vi "Configure.vi"(8 "error in (no error)":errorcluster caption="错误输入（无错误）", 11 "34401A 输入":refnum<class "34401A.lvclass">) -> (0 "error out":errorcluster caption="错误输出", 3 "34401A 输出":refnum<class "34401A.lvclass">)   [LabVIEW 2020, in "34401A.lvlib" / "34401A.lvclass"]
uses:
  34401A.lvclass
  <instrlib>/Agilent 34401/Agilent 34401.lvlib
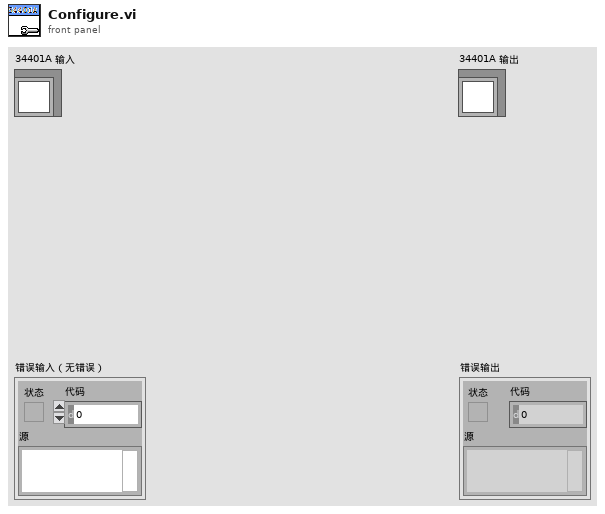
[diagram p1: front panel]
types:
  T1 = enum16{"DC Voltage", "AC Voltage", "Resistance", "DC Current", "AC Current"}
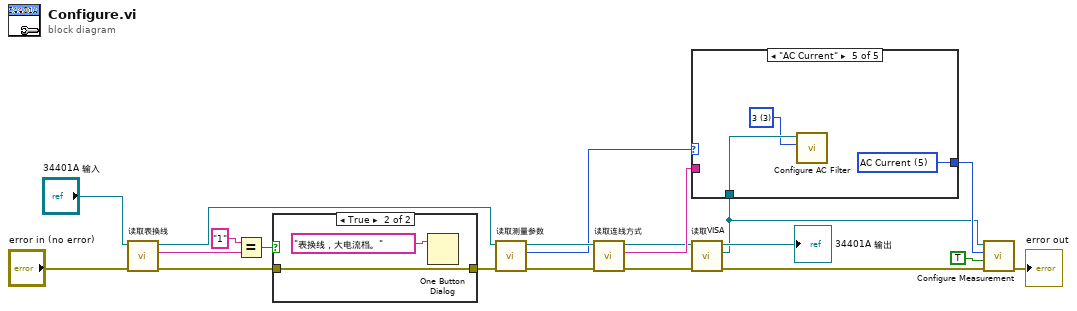
[diagram p0: block diagram]
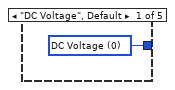
[diagram p3: hidden frame]
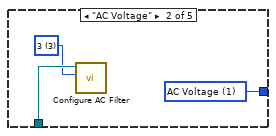
[diagram p4: hidden frame]
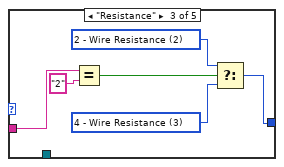
[diagram p5: hidden frame]
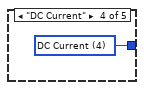
[diagram p6: hidden frame]
diagram:
  n1 = call "读取表换线.vi"("error in (no error)"="error in (no error)", "数字多用表接口输入"="34401A 输入") -> ("error out"=w3:errorcluster, "表换线"=w5:string, "数字多用表接口输出"=w7:refnum<class "34401A.lvclass">)  [unwired: 7 in]
  n2 = Equal?(x="1" ("y"), y=w5) -> (x = y?=w4:bool)
  n3 = case shown="True" w4 {
    tunnel: w3 -> [w21 w22]
    tunnel: [w21 w22] -> w2
    frame False {
    }
    frame True {
      n4 = One Button Dialog(message="表换线，大电流档。" ("消息")) -> ()  [unwired: 1 in, 1 out]
    }
  }
  n5 = call "读取测量参数.vi"("error in (no error)"=w2, "数字多用表接口输入"=w7) -> ("error out"=w17:errorcluster, "测量参数"=w16:T1, "数字多用表接口输出"=w19:refnum<class "34401A.lvclass">)  [unwired: 7 in]
  n6 = call "读取连线方式.vi"("error in (no error)"=w17, "数字多用表接口输入"=w19) -> ("error out"=w14:errorcluster, "连线方式"=w18:string, "数字多用表接口输出"=w15:refnum<class "34401A.lvclass">)  [unwired: 7 in]
  n7 = call "读取VISA.vi"("error in (no error)"=w14, "数字多用表接口输入"=w15) -> ("error out"=w12:errorcluster, "VISA"=w1:refnum<visa-resource-name>, "数字多用表接口输出"=→"34401A 输出":refnum<class "34401A.lvclass">)  [unwired: 7 in]
  n8 = case shown="\"AC Current\"" w16 {
    tunnel: [w24 w27 w28 w34 w37] -> w20
    tunnel: w18 -> [_ _ w29 _ _]
    tunnel: w1 -> [_ w26 _ _ w36]
    frame "DC Voltage", Default {
      w24 = u16 0 items=["DC Voltage", "AC Voltage", "2 - Wire Resistance", "4 - Wire Resistance", "DC Current", "AC Current", "Frequency", "Period", "Continuity", "Diode Checking", "VDC:VDC Ratio", "Temperature", "Capacitance"] ("Function (0: DC Voltage)")
    }
    frame "AC Voltage" {
      w25 = 3 items=["3"=3, "20"=20, "200"=200] ("AC Filter Bandwidth (20 Hz)")
      w27 = u16 1 items=["DC Voltage", "AC Voltage", "2 - Wire Resistance", "4 - Wire Resistance", "DC Current", "AC Current", "Frequency", "Period", "Continuity", "Diode Checking", "VDC:VDC Ratio", "Temperature", "Capacitance"] ("Function (0: DC Voltage)")
      n9 = call <instrlib>:"Configure AC Filter.vi"("AC Filter Bandwidth (20 Hz)"=w25, "VISA resource name"=w26) -> ()  [unwired: 8 in, 2 out]
    }
    frame "Resistance" {
      w33 = u16 3 items=["DC Voltage", "AC Voltage", "2 - Wire Resistance", "4 - Wire Resistance", "DC Current", "AC Current", "Frequency", "Period", "Continuity", "Diode Checking", "VDC:VDC Ratio", "Temperature", "Capacitance"] ("Function (0: DC Voltage)")
      w32 = u16 2 items=["DC Voltage", "AC Voltage", "2 - Wire Resistance", "4 - Wire Resistance", "DC Current", "AC Current", "Frequency", "Period", "Continuity", "Diode Checking", "VDC:VDC Ratio", "Temperature", "Capacitance"] ("Function (0: DC Voltage)")
      n10 = Equal?(x=w29, y="2") -> (x = y?=w31:bool)
      n11 = Select(t=w32, s=w31, f=w33) -> (s? t:f=w28:u16)
    }
    frame "DC Current" {
      w34 = u16 4 items=["DC Voltage", "AC Voltage", "2 - Wire Resistance", "4 - Wire Resistance", "DC Current", "AC Current", "Frequency", "Period", "Continuity", "Diode Checking", "VDC:VDC Ratio", "Temperature", "Capacitance"] ("Function (0: DC Voltage)")
    }
    frame "AC Current" {
      w35 = 3 items=["3"=3, "20"=20, "200"=200] ("AC Filter Bandwidth (20 Hz)")
      w37 = u16 5 items=["DC Voltage", "AC Voltage", "2 - Wire Resistance", "4 - Wire Resistance", "DC Current", "AC Current", "Frequency", "Period", "Continuity", "Diode Checking", "VDC:VDC Ratio", "Temperature", "Capacitance"] ("Function (0: DC Voltage)")
      n12 = call <instrlib>:"Configure AC Filter.vi"("AC Filter Bandwidth (20 Hz)"=w35, "VISA resource name"=w36) -> ()  [unwired: 8 in, 2 out]
    }
  }
  n13 = call <instrlib>:"Configure Measurement.vi"("error in (no error)"=w12, "Enable Auto Range (T: Enable)"=TRUE, "Function (0: DC Voltage)"=w20, "VISA resource name"=w1) -> ("error out"=→"error out":errorcluster)  [unwired: 6 in, 1 out]
